vi "Function_Block Spot.vi"(0 "Image Dst In":T4, 5 "Data Cluster In":cluster{"Name":string, "Variant In":variant}, 7 "CoordSys In":T1 {"Measurement System"."Axis Reference" items=["Direct", "Indirect"]; "Measurement System"."Angle (deg)" format="%.2f"; "Measurement System"."Origin"."Y" format="%.2f"; "Measurement System"."Origin"."X" format="%.2f"; "Reference System"."Axis Reference" items=["Direct", "Indirect"]; "Reference System"."Angle (deg)" format="%.2f"; "Reference System"."Origin"."Y" format="%.2f"; "Reference System"."Origin"."X" format="%.2f"}, 9 "Center(Annulus)":cluster{"X":sgl, "Y":sgl} {"Y" format="%.2f"; "X" format="%.2f"}, 11 "Error in":errorcluster) -> (4 "Objects":T3(array[cluster]) {"Area" format="%.2f"; "Object Center"."Y" format="%.2f"; "Object Center"."X" format="%.2f"}, 6 "Result(Black)":cluster{"Name":string, "NG?":bool, "Score":dbl}, 10 "ROI Out":T2 {"Contours"."Type" items=["No Selection", "Point", "Line", "Rectangle", "Oval", "Polygon", "Free", "Annulus", "Unused2", "Unused3", "Broken Line", "Free Hand Line", "Rotated Rectangle"]}, 14 "Time":u32, 15 "Error out":errorcluster)   [LabVIEW 2013]
uses:
  <vilib>/vision/Image Controls.llb/IMAQ Image.ctl
  Control/Control_Block Spot.ctl
  <vilib>/vision/NI_Vision_Development_Module.lvlib
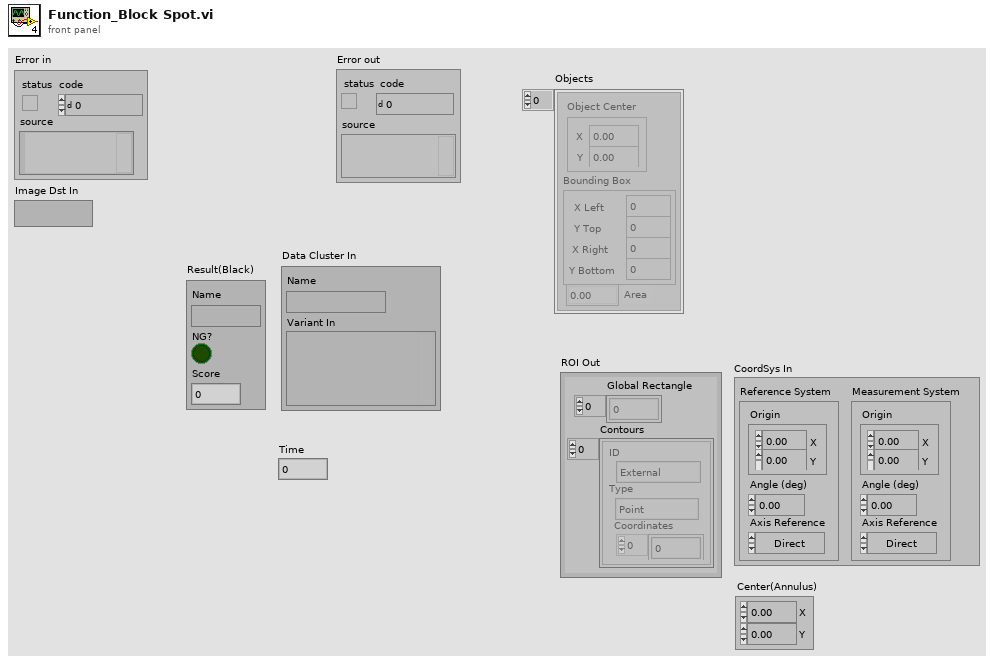
[diagram p1: front panel]
types:
  T1 = typedef "IMAQ Coordinate System" = cluster{"Reference System":cluster{"Origin":cluster{"X":sgl, "Y":sgl}, "Angle (deg)":sgl, "Axis Reference":u32}, "Measurement System":cluster{"Origin":cluster{"X":sgl, "Y":sgl}, "Angle (deg)":sgl, "Axis Reference":u32}}
  T2 = cluster{"Global Rectangle":i32[], "Contours":cluster{"ID":enum32{"External", "Internal"}, "Type":u32, "Coordinates":i32[]}[]}
  T3 = cluster{"Object Center":cluster{"X":dbl, "Y":dbl}, "Bounding Box":cluster{"X Left":dbl, "Y Top":dbl, "X Right":dbl, "Y Bottom":dbl}, "Area":dbl}[]
  T4 = typedef "IMAQ Image.ctl" = refnum<image>
  T5 = typedef "Control_Block Spot.ctl" = cluster{"Name":string, "ROI":cluster{"Global Rectangle":i32[], "Contours":cluster{"ID":enum32{"External", "Internal"}, "Type":u32, "Coordinates":i32[]}[]}, "Magnification(黑點)":i32, "Settings(黑點)":cluster{"Objects":enum16{"Bright Objects", "Dark Objects"}, "Threshold":i32, "Min Object Size":bool, "Min Size":i32, "Max Object Size":bool, "Max Size":i32}, "Highlight":cluster{"Kernel Size":i32, "Divider":sgl, "Min Object Size":bool}}
  T6 = cluster{"Objects":enum16{"Bright Objects", "Dark Objects"}, "Threshold":i32, "Min Object Size":bool, "Min Size":i32, "Max Object Size":bool, "Max Size":i32}
  T7 = cluster{"Kernel Size":i32, "Divider":sgl, "Min Object Size":bool}
  T8 = cluster{"ID":enum32{"External", "Internal"}, "Type":u32, "Coordinates":i32[]}[]
  T9 = cluster{"ID":enum32{"External", "Internal"}, "Type":u32, "Coordinates":i32[]}
  T10 = cluster{"Origin":cluster{"X":sgl, "Y":sgl}, "Angle (deg)":sgl, "Axis Reference":u32}
  T11 = typedef "ROI Descriptor" = cluster{"Global Rectangle":i32[], "Contours":cluster{"ID":enum32{"External", "Internal"}, "Type":u32, "Coordinates":i32[]}[]}
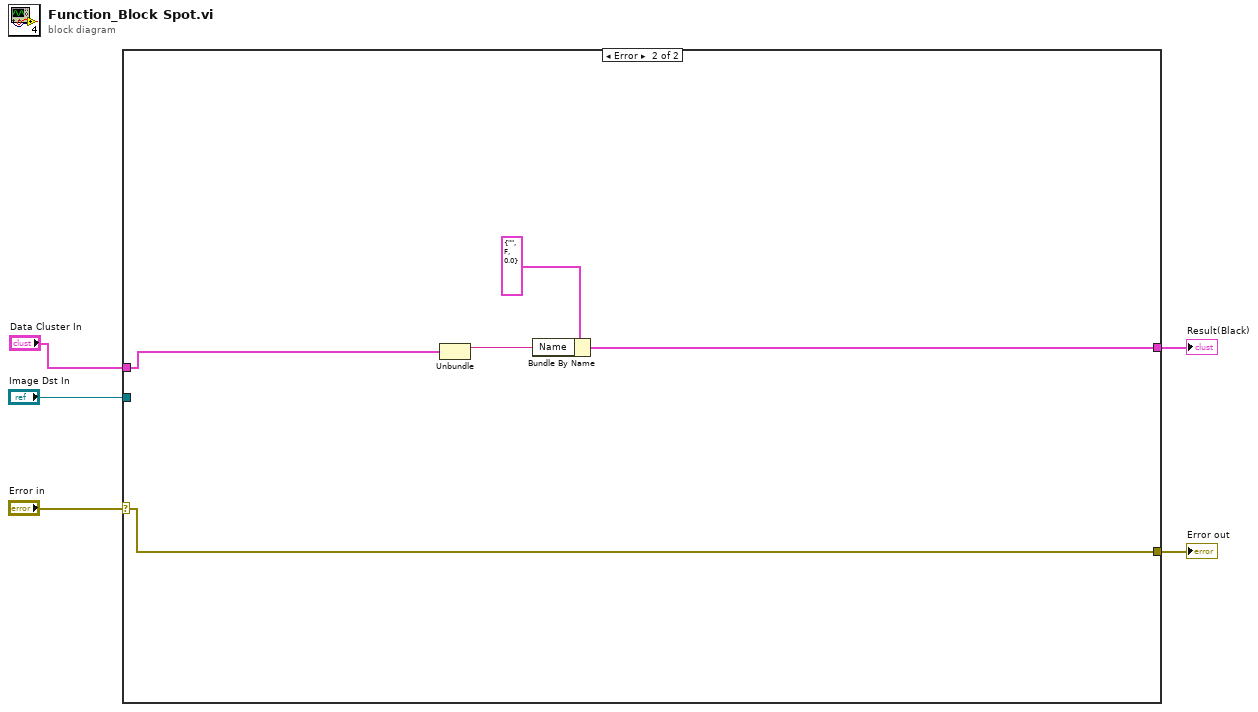
[diagram p0: block diagram]
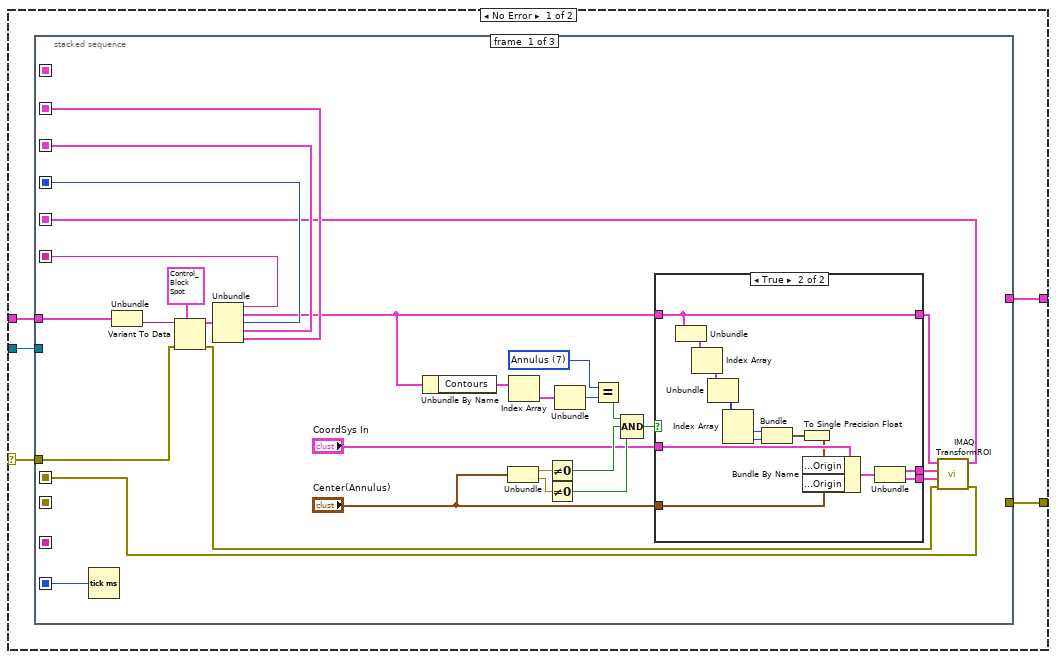
[diagram p2: hidden frame]
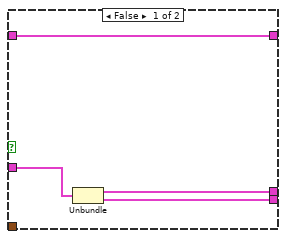
[diagram p3: hidden frame]
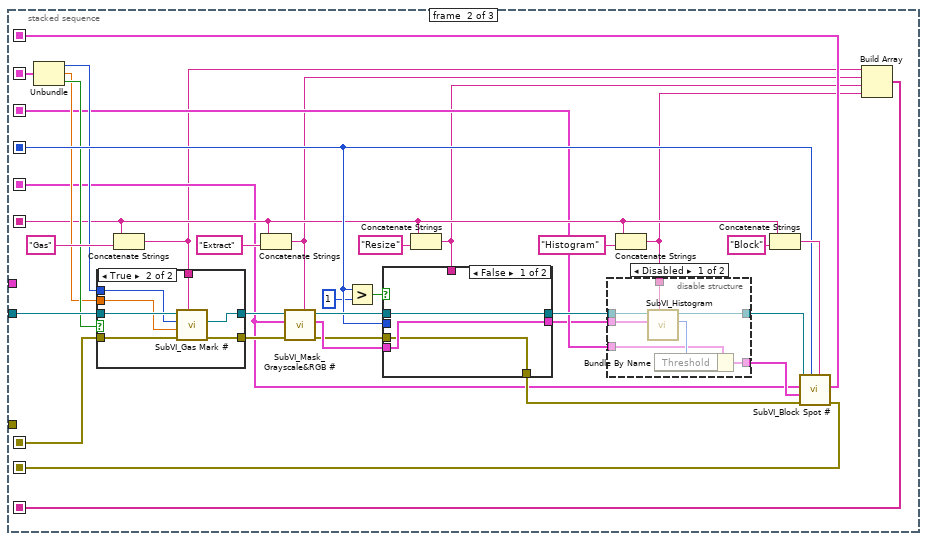
[diagram p4: hidden frame]
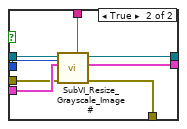
[diagram p7: hidden frame]
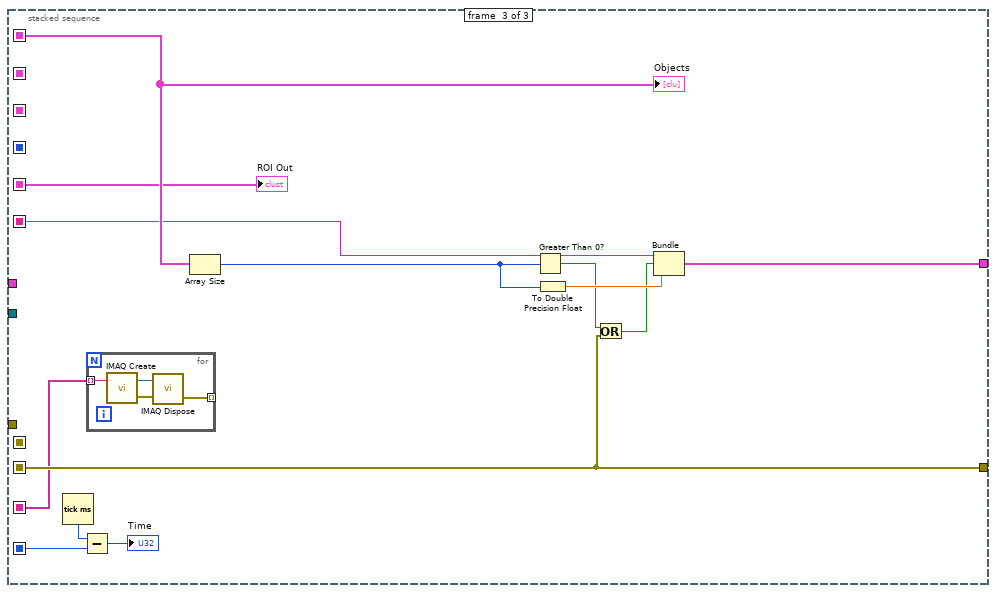
[diagram p8: hidden frame]
diagram:
  n1 = case shown="Error" "Error in" {
    selector: "Error in" -> [w7 w142]
    tunnel: [w10 w142] -> w5
    tunnel: "Image Dst In" -> [w9 _]
    tunnel: [w8 w138] -> w3
    tunnel: "Data Cluster In" -> [w6 w139]
    frame No Error {
      n2 = stacked-sequence {
        seq-local: [w37 _ _] -> [_ w70 w127]
        seq-local: [w16 _ _] -> [_ w68 w125]
        seq-local: [w36 _ _] -> [_ w81 _]
        seq-local: [w35 _ _] -> [_ w69 _]
        seq-local: [w34 _ _] -> [_ _ w131]
        seq-local: [w33 _ _] -> [_ w79 _]
        seq-local: [_ w62 _] -> [_ _ w122]
        seq-local: [_ w65 _] -> [_ _ w130]
        seq-local: [w12 _ _] -> [_ w64 _]
        seq-local: [_ w57 _] -> [_ _ w121]
        tunnel: [_ _ w122] -> w10
        tunnel: w7 -> [w15 _ _]
        tunnel: w9 -> [_ w84 _]
        tunnel: [_ _ w126] -> w8
        tunnel: w6 -> [w11 _ _]
        frame #0 {
          w21 = u32 7 items=["No Selection", "Point", "Line", "Rectangle", "Oval", "Polygon", "Freehand Region", "Annulus", "Unused2", "Unused3", "Broken Line", "Freehand Line", "Rotated Rectangle"] ("Type")
          n3 = Tick Count (ms)() -> (millisecond timer value=w34:u32)
          n4 = Unbundle(w11) -> ("Variant In"=w38:variant)  [unwired: 1 out]
          n5 = Variant To Data(error in=w15, type=T5 {"Name"="", "ROI"={"Global Rectangle"=[], "Contours"=[]}, "Magnification(黑點)"=0, "Settings(黑點)"={"Objects"=enum."Bright Objects", "Threshold"=0, "Min Object Size"=FALSE, "Min Size"=0, "Max Object Size"=FALSE, "Max Size"=0}, "Highlight"={"Kernel Size"=0, "Divider"=0.0, "Min Object Size"=FALSE}} ("黑點_Setting"), Variant=w38) -> (data=w39:T5, error out=w14:errorcluster)
          n6 = Unbundle(w39) -> ("Name"=w37:string, "ROI"=w17:T2, "Magnification(黑點)"=w36:i32, "Settings(黑點)"=w35:T6, "Highlight"=w33:T7)
          n7 = Unbundle By Name(w17) -> ("Contours"=w23:T8)
          n8 = Unbundle("Center(Annulus)") -> ("X"=w27:sgl, "Y"=w28:sgl)
          n9 = Index Array(array=w23) -> (element=w22:T9)  [unwired: 1 in]
          n10 = Not Equal To 0?(x=w27) -> (x != 0?=w30:bool)
          n11 = Not Equal To 0?(x=w28) -> (x != 0?=w31:bool)
          n12 = Unbundle(w22) -> ("Type"=w20:u32)  [unwired: 2 out]
          n13 = Equal?(x=w21, y=w20) -> (x = y?=w29:bool)
          n14 = Compound Arithmetic op=AND(w29, w30, w31) -> (w32:bool)
          n15 = case shown="True" w32 {
            tunnel: "CoordSys In" -> [w43 w56]
            tunnel: [w42 w50] -> w19
            tunnel: [w41 w49] -> w18
            tunnel: "Center(Annulus)" -> [_ w53]
            tunnel: w17 -> [w40 w44]
            tunnel: [w40 w44] -> w25
            frame False {
              n16 = Unbundle(w43) -> ("Reference System"=w42:T10, "Measurement System"=w41:T10)
            }
            frame True {
              n17 = Unbundle(w44) -> ("Contours"=w48:T8)  [unwired: 1 out]
              n18 = Index Array(array=w48) -> (element=w47:T9)  [unwired: 1 in]
              n19 = Unbundle(w47) -> ("Coordinates"=w46:i32[])  [unwired: 2 out]
              n20 = Index Array(array=w46) -> (element #1=w55:i32, element #2=w54:i32)  [unwired: 2 in]
              n21 = Bundle(w55, w54) -> (w45:cluster{i32, i32})  [unwired: 1 in]
              n22 = To Single Precision Float(number=w45) -> (single precision float=w52:cluster{sgl, sgl})
              n23 = Bundle By Name(cluster=w56, "Reference System.Origin"=w52, "Measurement System.Origin"=w53) -> (w51:T1)
              n24 = Unbundle(w51) -> ("Reference System"=w50:T10, "Measurement System"=w49:T10)
            }
          }
          n25 = call "IMAQ TransformROI"("error in (no error)"=w14, "New Reference"=w18, "Base Reference"=w19, "ROI Descriptor"=w25) -> ("error out"=w12:errorcluster, "ROI Descriptor out"=w16:T11)  [unwired: 6 in]
        }
        frame #1 {
          n26 = Unbundle(w79) -> ("Kernel Size"=w77:i32, "Divider"=w76:sgl, "Min Object Size"=w78:bool)
          n27 = Concatenate Strings(w70, "Gas" ("string")) -> (w61:string)
          n28 = case shown="True" w78 {
            tunnel: w84 -> [w102 w109]
            tunnel: [w102 w108] -> w83
            tunnel: w61 -> [_ w107]
            tunnel: w77 -> [_ w106]
            tunnel: w76 -> [_ w105]
            tunnel: w64 -> [w101 w104]
            tunnel: [w101 w103] -> w75
            frame False {
            }
            frame True {
              n29 = call "SubVI_Gas Mark #.vi"("Image Register Name"=w107, "Error in"=w104, "Divider"=w105, "Kernel Size"=w106, "Image Src In"=w109) -> ("Error out"=w103:errorcluster, "Image Dst Out"=w108:T4)  [unwired: 4 in, 1 out]
            }
          }
          n30 = Concatenate Strings(w70, "Extract" ("Image Register Name")) -> (w60:string)
          n31 = call "SubVI_Mask_Grayscale&RGB #.vi"("Image Register Name"=w60, "Error in"=w75, "ROI Descriptor"=w68, "Image Src In"=w83) -> ("Error out"=w63:errorcluster, "ROI Descriptor out"=w67:T11, "Image Dst Out"=w91:T4)  [unwired: 4 in, 1 out]
          n32 = Greater?(x=w81, y=1) -> (0:w82:bool)
          n33 = Concatenate Strings(w70, "Resize" ("Image Register Name")) -> (w59:string)
          n34 = case shown="False" w82 {
            tunnel: w91 -> [w112 w120]
            tunnel: w81 -> [_ w119]
            tunnel: w59 -> [_ w118]
            tunnel: [w110 w113] -> w86
            tunnel: [w112 w117] -> w72
            tunnel: w67 -> [w111 w116]
            tunnel: [w111 w115] -> w66
            tunnel: w63 -> [w110 w114]
            frame False {
            }
            frame True {
              n35 = call "SubVI_Resize_Grayscale_Image #.vi"("Image Register Name"=w118, "Magnification"=w119, "Error In"=w114, "ROI Descriptor"=w116, "Image Src In"=w120) -> ("Error Out"=w113:errorcluster, "ROI Descriptor out"=w115:T11, "Image Dst Out"=w117:T4)  [unwired: 3 in, 1 out]
            }
          }
          n36 = Concatenate Strings(w70, "Histogram" ("string")) -> (w58:string)
          n37 = disable-structure shown="Disabled" {
            disable-tunnel: w58 -> [w98 _]
            disable-tunnel: [w97 w100] -> w73
            disable-tunnel: w72 -> [w96 w100]
            disable-tunnel: [w95 w99] -> w71
            disable-tunnel: w69 -> [w93 w99]
            disable-tunnel: w66 -> [w92 _]
            frame Disabled {
              n38 = call "SubVI_Histogram.vi"("Image Register Name"=w98, "ROI Descriptor"=w92, "Image Sorce In"=w96) -> ("Mean Value"=w94:i32, "Image Sorce Out"=w97:T4)  [unwired: 6 in, 1 out]
              n39 = Bundle By Name(cluster=w93, "Threshold"=w94) -> (w95:T6)
            }
            frame Enabled {
            }
          }
          n40 = Concatenate Strings(w70, "Block" ("string")) -> (w88:string)
          n41 = call "SubVI_Block Spot #.vi"("Image Register Name"=w88, "Magnification"=w81, "Error in"=w86, "Settings"=w71, "ROI Descriptor"=w68, "Image Src In"=w73) -> ("Error out"=w62:errorcluster, "Objects"=w65:T3)  [unwired: 3 in, 1 out]
          n42 = Build Array(w61, w60, w59, w58) -> (w57:string[])
        }
        frame #2 {
          n43 = Tick Count (ms)() -> (millisecond timer value=w133:u32)
          n44 = Subtract(x=w133, y=w131) -> (x-y=→"Time":u32)
          n45 = for {
            tunnel: w121 -> [w137] mode=indexing
            tunnel: [w134] -> _ mode=indexing
            n46 = call "IMAQ Create"("Image Name"=w137) -> ("New Image"=w136:T4, "error out"=w135:errorcluster)  [unwired: 4 in]
            n47 = call "IMAQ Dispose"("Image"=w136, "error in (no error)"=w135) -> ("error out"=w134:errorcluster)  [unwired: 4 in]
          }
          n48 = Array Size(array=w130) -> (size(s)=w128:i32)
          n49 = Greater Than 0?(x=w128) -> (x > 0?=w124:bool)
          n50 = To Double Precision Float(number=w128) -> (double precision float=w129:dbl)
          n51 = Or(x=w124, y=w122) -> (x .or. y?=w123:bool)
          n52 = Bundle("Name"=w127, w123, w129) -> (w126:cluster{"Name":string, bool, dbl})  [unwired: 1 in]
          "Objects" <- w130
          "ROI Out" <- w125
        }
      }
    }
    frame Error {
      n53 = Unbundle(w139) -> ("Name"=w140:string)  [unwired: 1 out]
      n54 = Bundle By Name(cluster=cluster{"Name":string, bool, "Radius":dbl} {"Name"="", FALSE, "Radius"=0.0}, "Name"=w140) -> (w138:cluster{"Name":string, bool, "Radius":dbl})
    }
  }
  "Error out" <- w5
  "Result(Black)" <- w3
